vi "NewMessageToSend.vi"(8 "error in (no error)":errorcluster, 9 "Connection Number":i32, 10 "Message":string, 11 "TCP_Server in":refnum<class "TCP_Server.lvclass">) -> (0 "error out":errorcluster, 3 "TCP_Server out":refnum<class "TCP_Server.lvclass">)   [LabVIEW 2023, in "TCP_Server.lvlib" / "TCP_Server.lvclass"]
uses:
  TCP_Server.lvclass
  TCP_Server.lvclass/TCP_Server.ctl
  TCP_Server_Connection_Handler/TCP_Server_Connection_Handler Messages/SendString Msg/SendString Msg.lvclass
  <vilib>/ActorFramework/Message Enqueuer/Message Enqueuer.lvclass
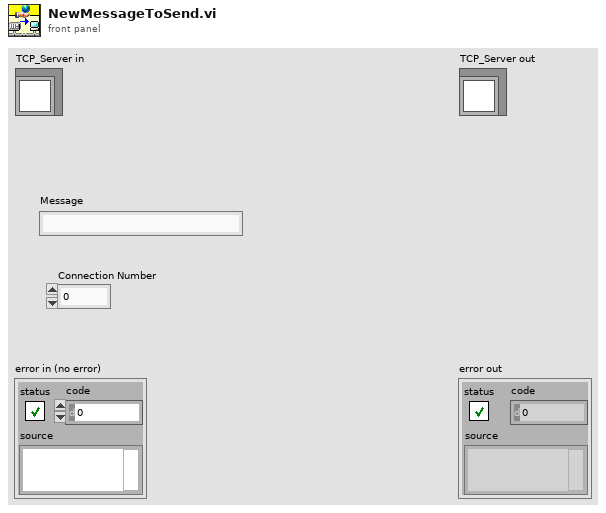
[diagram p1: front panel]
types:
  T1 = cluster{"Connection number":i32, "Remote Address":string, "Remote Port":u16, "Connection ID":refnum<k5>, "Connection Handlers's Enqueuer":refnum<class "Message Enqueuer.lvclass">, "Connection Window's Enqueuer":refnum<class "Message Enqueuer.lvclass">}[]
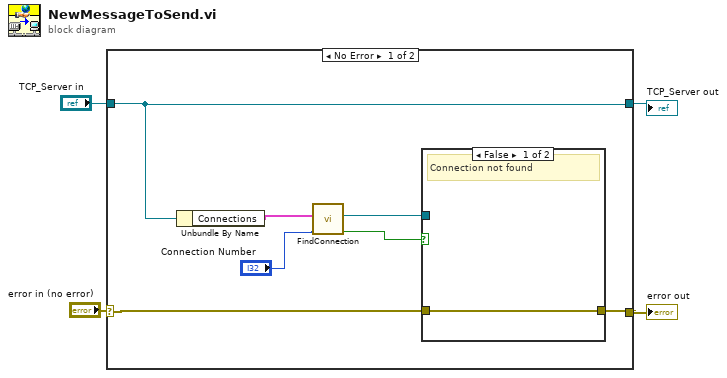
[diagram p0: block diagram]
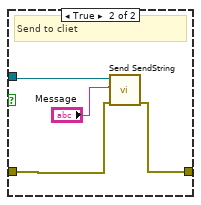
[diagram p2: hidden frame]
diagram:
  n1 = case shown="No Error" "error in (no error)" {
    selector: "error in (no error)" -> [w8 w18]
    tunnel: [w7 w18] -> w3
    tunnel: [w6 w17] -> w2
    tunnel: "TCP_Server in" -> [w6 w17]
    frame No Error {
      n2 = Unbundle By Name(w6) -> ("Connections"=w11:T1)
      n3 = call "FindConnection.vi"("Connection number"="Connection Number", "Connections"=w11) -> ("Found?"=w10:bool, "Connection Handlers's Enqueuer"=w9:refnum<class "Message Enqueuer.lvclass">)  [unwired: 6 in, 2 out]
      n4 = case shown="False" w10 {
        tunnel: w9 -> [_ w16]
        tunnel: w8 -> [w12 w14]
        tunnel: [w12 w13] -> w7
        frame False {
          # "Connection not found"
        }
        frame True {
          # "Send to cliet"
          n5 = call "Send SendString.vi"("error in (no error)"=w14, "Message"="Message", "Message Enqueuer"=w16) -> ("error out"=w13:errorcluster)  [unwired: 7 in, 1 out]
        }
      }
    }
    frame Error {
    }
  }
  "error out" <- w3
  "TCP_Server out" <- w2
